vi "SettingCamera.vi"(8 "error in (no error)":errorcluster, 9 "Value":dbl, 10 "Label":string, 11 "Microscope in":refnum<class "Microscope.lvclass">) -> (0 "error out":errorcluster, 3 "Microscope out":refnum<class "Microscope.lvclass">)   [LabVIEW 2020, in "Microscope.lvlib" / "Microscope.lvclass"]
uses:
  Microscope.lvclass
  Microscope.lvclass/Microscope.ctl
  Component/Camera/Camera Messages/SetExposure Msg/SetExposure Msg.lvclass/SetExposure Msg.ctl
  <vilib>/ActorFramework/Message Enqueuer/Message Enqueuer.lvclass/Message Enqueuer.ctl
  Component/Camera/Camera Messages/SetFrameToCaptureNumber Msg/SetFrameToCaptureNumber Msg.lvclass/SetFrameToCaptureNumber Msg.ctl
  Component/Camera/Camera Messages/SetInterval Msg/SetInterval Msg.lvclass/SetInterval Msg.ctl
  <vilib>/ActorFramework/Message Enqueuer/Enqueue.vi
  Component/Camera/Camera Messages/SetExposure Msg/SetExposure Msg.lvclass
  C:/Program Files/National Instruments/LabVIEW 2020/vi.lib/ActorFramework/Message/Message.lvclass
  Component/Camera/Camera Messages/SetFrameToCaptureNumber Msg/SetFrameToCaptureNumber Msg.lvclass
  Component/Camera/Camera Messages/SetInterval Msg/SetInterval Msg.lvclass
  <vilib>/ActorFramework/Message Priority Queue/Priority Enqueue.vi
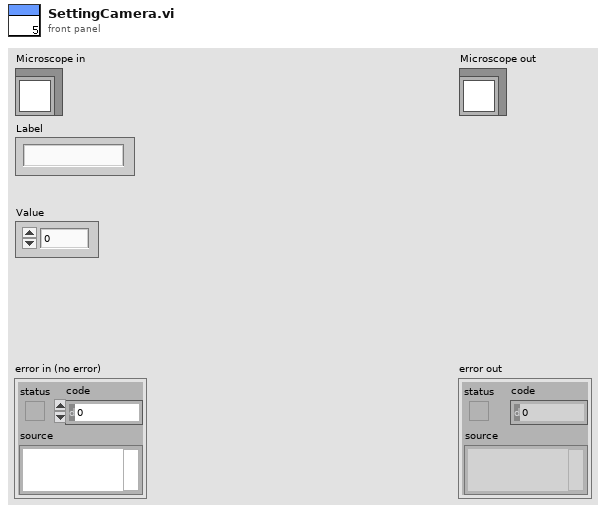
[diagram p1: front panel]
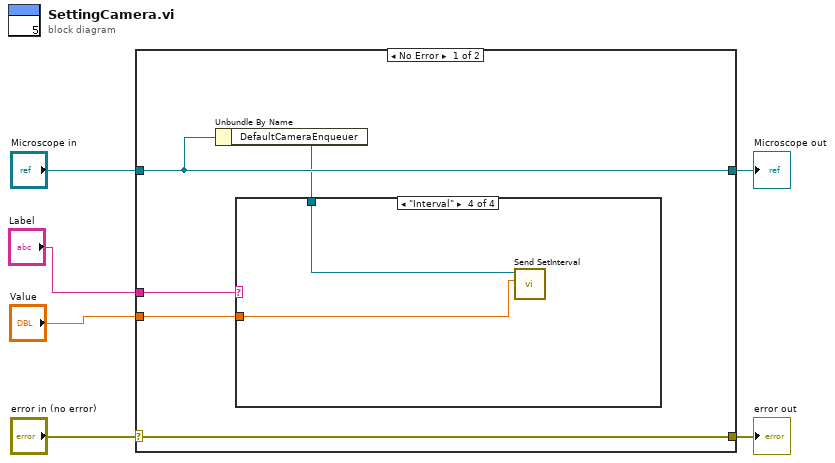
[diagram p0: block diagram]
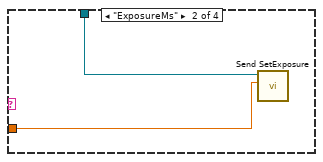
[diagram p3: hidden frame]
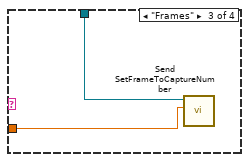
[diagram p4: hidden frame]
diagram:
  n1 = case shown="No Error" "error in (no error)" {
    selector: "error in (no error)" -> [w11 w19]
    tunnel: [w11 w19] -> w5
    tunnel: [w8 w18] -> w3
    tunnel: "Microscope in" -> [w8 w18]
    tunnel: "Value" -> [w10 _]
    tunnel: "Label" -> [w9 _]
    frame No Error {
      n2 = Unbundle By Name(w8) -> ("DefaultCameraEnqueuer"=w7:refnum<class "Message Enqueuer.lvclass">)
      n3 = case shown="\"Interval\"" w9 {
        tunnel: w10 -> [_ w12 w14 w16]
        tunnel: w7 -> [_ w13 w15 w17]
        frame Default {
        }
        frame "ExposureMs" {
          n4 = call "Send SetExposure.vi"("Setting.Exposure"=w12, "Message Enqueuer"=w13) -> ()  [unwired: 8 in, 2 out]
        }
        frame "Frames" {
          n5 = call "Send SetFrameToCaptureNumber.vi"("Setting.FramesToCapture"=w14, "Message Enqueuer"=w15) -> ()  [unwired: 8 in, 2 out]
        }
        frame "Interval" {
          n6 = call "Send SetInterval.vi"("Setting.Interval"=w16, "Message Enqueuer"=w17) -> ()  [unwired: 8 in, 2 out]
        }
      }
    }
    frame Error {
    }
  }
  "error out" <- w5
  "Microscope out" <- w3
